vi "svfa_Average Array with Avg Checks (complex) (1 Ch).vi"(0 "spectrum":cdb[](array[numeric]) format="%.2p", 1 "processing control":T1(ring), 7 "averaging parameters":T2={"averaging mode"=enum."No averaging", "weighting mode"=enum."Linear", "number of averages"=10, "linear mode"=enum."Auto restart"}, 11 "error in (no error)":errorcluster) -> (4 "average spectrum":cdb[](array[numeric]) format="%.2p", 6 "new spectrum ready":bool, 8 "averaging done":bool, 10 "averages completed":dbl, 15 "error out":errorcluster)   [LabVIEW 2017]
uses:
  <vilib>/addons/_NISVFA/_Shared subVIs/Spectrum Averaging/svfa_Average Array (complex) No State.vi
  <vilib>/addons/_NISVFA/_Shared subVIs/Spectrum Averaging/svfa_No Average Array (complex).vi
  <vilib>/addons/_NISVFA/_Shared subVIs/Spectrum Averaging/svfa_Average Array (complex).vi
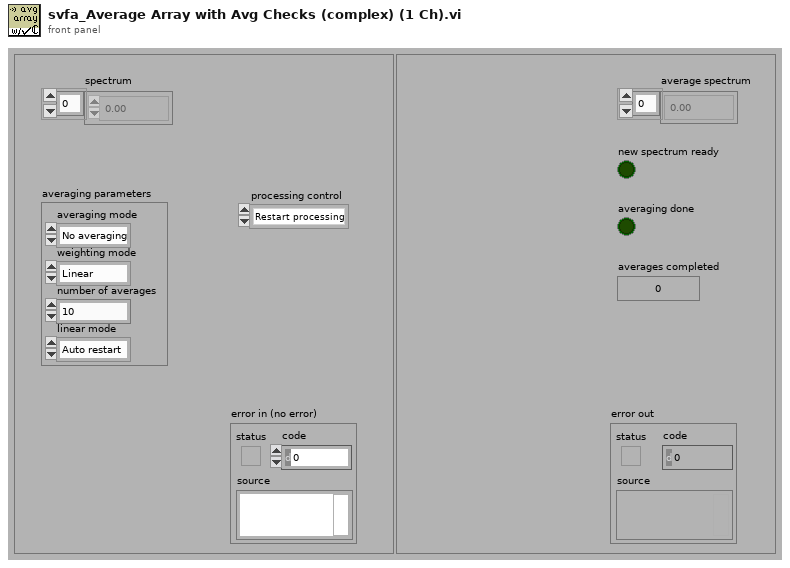
[diagram p1: front panel]
types:
  T1 = enum16{"Restart processing", "Continue processing", "Skip processing"}
  T2 = cluster{"averaging mode":enum16{"No averaging", "Vector averaging", "RMS averaging", "Peak hold"}, "weighting mode":enum16{"Linear", "Exponential"}, "number of averages":u32, "linear mode":enum16{"One shot", "Auto restart"}}
  T3 = cluster{"complex FFT":cdb[], "real FFT":dbl[], "f0":dbl, "df":dbl, "averages completed":dbl, "averaging parameters":cluster{"averaging mode":enum16{"No averaging", "Vector averaging", "RMS averaging", "Peak hold"}, "weighting mode":enum16{"Linear", "Exponential"}, "number of averages":u32, "linear mode":enum16{"One shot", "Auto restart"}}}
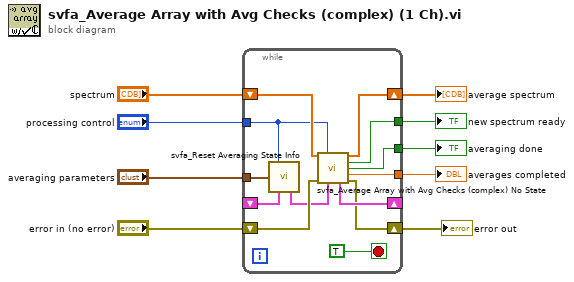
[diagram p0: block diagram]
diagram:
  n1 = while {
    tunnel: "processing control" -> [w10]
    shift-left: _ -> [w12]
    shift-right: [w17] -> _
    tunnel: [w14] -> w4
    tunnel: [w19] -> w5
    tunnel: [w20] -> w6
    tunnel: "averaging parameters" -> [w13]
    shift-right: [w21] -> w7
    shift-left: "spectrum" -> [w22]
    shift-right: [w15] -> w3
    shift-left: "error in (no error)" -> [w16]
    stop <- TRUE stop-if-true
    n2 = call <vilib>:"svfa_Reset Averaging State Info.vi"("processing control"=w10, "averaging parameters"=w13, "averaging state info in"=w12) -> ("averaging state info out"=w11:T3)  [unwired: 11 in, 1 out]
    n3 = call <vilib>:"svfa_Average Array with Avg Checks (complex) No State.vi"("spectrum"=w22, "processing control"=w10, "error in (no error)"=w16, "averaging state info in"=w11) -> ("average spectrum"=w21:cdb[], "new spectrum ready"=w20:bool, "averaging done"=w19:bool, "averages completed"=w14:dbl, "averaging state info out"=w17:T3, "error out"=w15:errorcluster)  [unwired: 6 in]
  }
  "average spectrum" <- w7
  "averages completed" <- w4
  "new spectrum ready" <- w6
  "averaging done" <- w5
  "error out" <- w3
